vi "Settings Dialog.vi"(8 "error in (no error)":errorcluster, 11 "Settings in":T3={"Connection Configuration"={"Data source"=enum."Serial port", "Connection info"={"VISA resource name"="COM 1", "Baud rate"=9600, "data bits"=8, "stop bits"=0, "parity (0:none)"=enum."None", "flow control (0:none)"=0, "timeout (10sec)"=10000, "termination char\n(0xA = '\\n' = LF) "=10, "Enable Termination\nChar (T)"=TRUE}, "Protocol info"={"Temination char"=255, "Escape char"=254}, "Internet server"={"Web page telemetry"="", "Web page gps"=""}, "Data format"=enum."IDRA data"}, "Logging Configuration"={"Log File Base Path"=path "", "TDMS File Reference"=refnum, "Data format"=enum."IDRA data"}, "Maps config"={"Real-time map config"={"Config path"=path "", "Image path"=path ""}, "Mini map config"={"Config path"=path "", "Image path"=path ""}}, "Data format"=enum."IDRA data"} {"Connection Configuration"."Connection info"."flow control (0:none)" items=["None", "XON/XOFF", "RTS/CTS", "XON/XOFF & RTS/CTS", "DTR/DSR", "XON/XOFF & DTR/DSR"]}) -> (0 "error out":errorcluster, 1 "Cancelled?":bool, 2 "UI Refresh Needed?":bool, 3 "Settings out":T3={"Connection Configuration"={"Data source"=enum."Serial port", "Connection info"={"VISA resource name"="COM 1", "Baud rate"=9600, "data bits"=8, "stop bits"=0, "parity (0:none)"=enum."None", "flow control (0:none)"=0, "timeout (10sec)"=10000, "termination char\n(0xA = '\\n' = LF) "=10, "Enable Termination\nChar (T)"=TRUE}, "Protocol info"={"Temination char"=255, "Escape char"=254}, "Internet server"={"Web page telemetry"="", "Web page gps"=""}, "Data format"=enum."IDRA data"}, "Logging Configuration"={"Log File Base Path"=path "", "TDMS File Reference"=refnum, "Data format"=enum."IDRA data"}, "Maps config"={"Real-time map config"={"Config path"=path "", "Image path"=path ""}, "Mini map config"={"Config path"=path "", "Image path"=path ""}}, "Data format"=enum."IDRA data"} {"Connection Configuration"."Connection info"."flow control (0:none)" items=["None", "XON/XOFF", "RTS/CTS", "XON/XOFF & RTS/CTS", "DTR/DSR", "XON/XOFF & DTR/DSR"]})   [LabVIEW 2015, in "Settings.lvlib"]
doc: "Dialog for selecting user specified settings."
uses:
  Settings.lvlib
  Settings.ctl
  Acquisition/Hardware Configuration.ctl
  Logging/Logging Configuration.ctl
  My Graphs/Gps Map Graph config.ctl
  <vilib>/Utility/xml.llb/Write to XML File(string).vi
  Acquisition/Acquisition.lvlib
  Logging/Logging.lvlib
panel:
  in  "Tab Control":T1(tab)
  in  "Web page gps":string
  in  "Web page telemetry":string
  in  "Data source":T2(ring)
  in  "Baud rate":u32=9600
  in  "Serial port":refnum<visa-resource-name>="COM 1"
  out "Previous data format":enum16{"IDRA data", "XAM data"}(ring)
  in  "Data format":enum16{"IDRA data", "XAM data"}(ring)
  in  "Folder for Log Files":path
  in  "Mini map image (350 x 200)":path
  in  "Configuration path":path
  in  "Big map image (780 x 550)":path
  in  "Cancel Button":bool
  in  "OK Button":bool
  # "Non visible portion of dialog (needed for connector pane)."
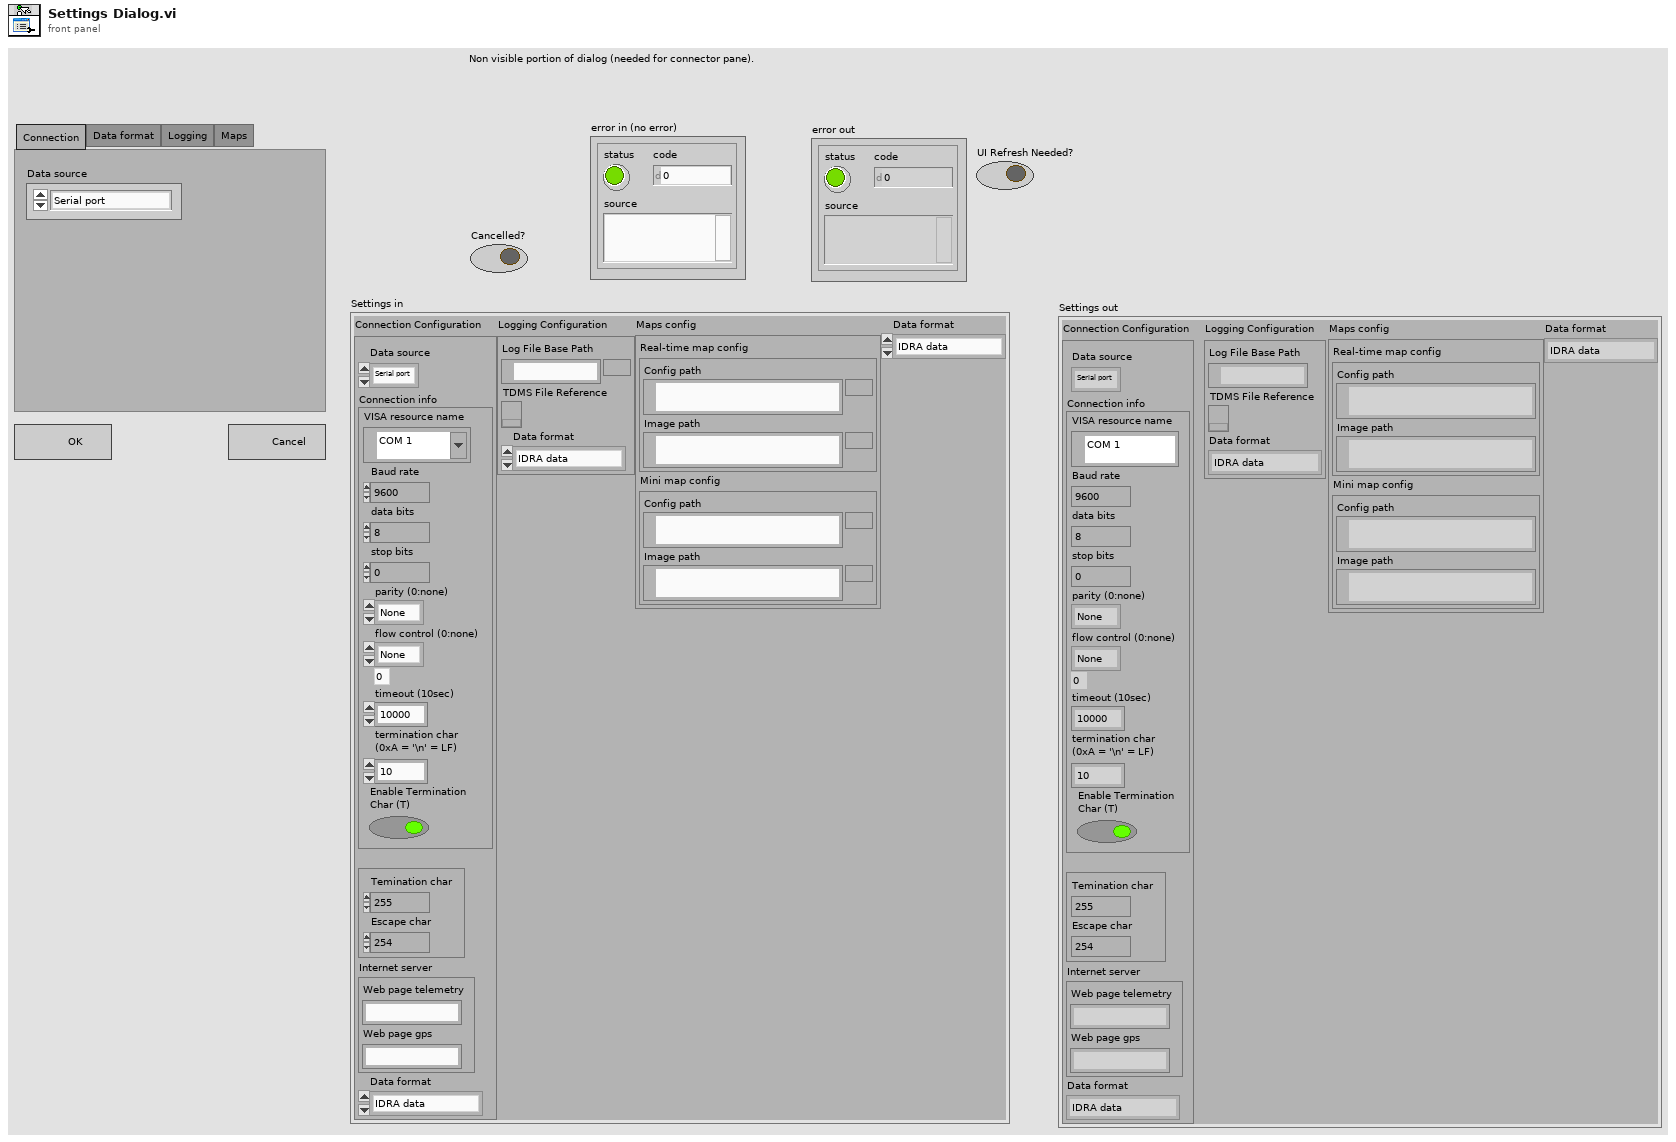
[diagram p1: front panel]
types:
  T1 = enum32{"Connection", "Data format", "Logging", "Maps"}
  T2 = enum16{"Serial port", "Simulated data", "Web page JSON"}
  T3 = typedef "Settings.lvlib/Settings.ctl" = cluster{"Connection Configuration":T4, "Logging Configuration":T5, "Maps config":cluster{"Real-time map config":T6, "Mini map config":T6}, "Data format":enum16{"IDRA data", "XAM data"}}
  T4 = typedef "Acquisition.lvlib/Hardware Configuration.ctl" = cluster{"Data source":enum16{"Serial port", "Simulated data", "Web page JSON"}, "Connection info":cluster{"VISA resource name":refnum<visa-resource-name>, "Baud rate":u32, "data bits":u16, "stop bits":u16, "parity (0:none)":enum16{"None", "Odd", "Even", "Mark", "Space"}, "flow control (0:none)":u16, "timeout (10sec)":u32, "termination char\n(0xA = '\\n' = LF) ":u8, "Enable Termination\nChar (T)":bool}, "Protocol info":cluster{"Temination char":u8, "Escape char":u8}, "Internet server":cluster{"Web page telemetry":string, "Web page gps":string}, "Data format":enum16{"IDRA data", "XAM data"}}
  T5 = typedef "Logging.lvlib/Logging Configuration.ctl" = cluster{"Log File Base Path":path, "TDMS File Reference":refnum<k34>, "Data format":enum16{"IDRA data", "XAM data"}}
  T6 = typedef "Gps Map Graph config.ctl" = cluster{"Config path":path, "Image path":path}
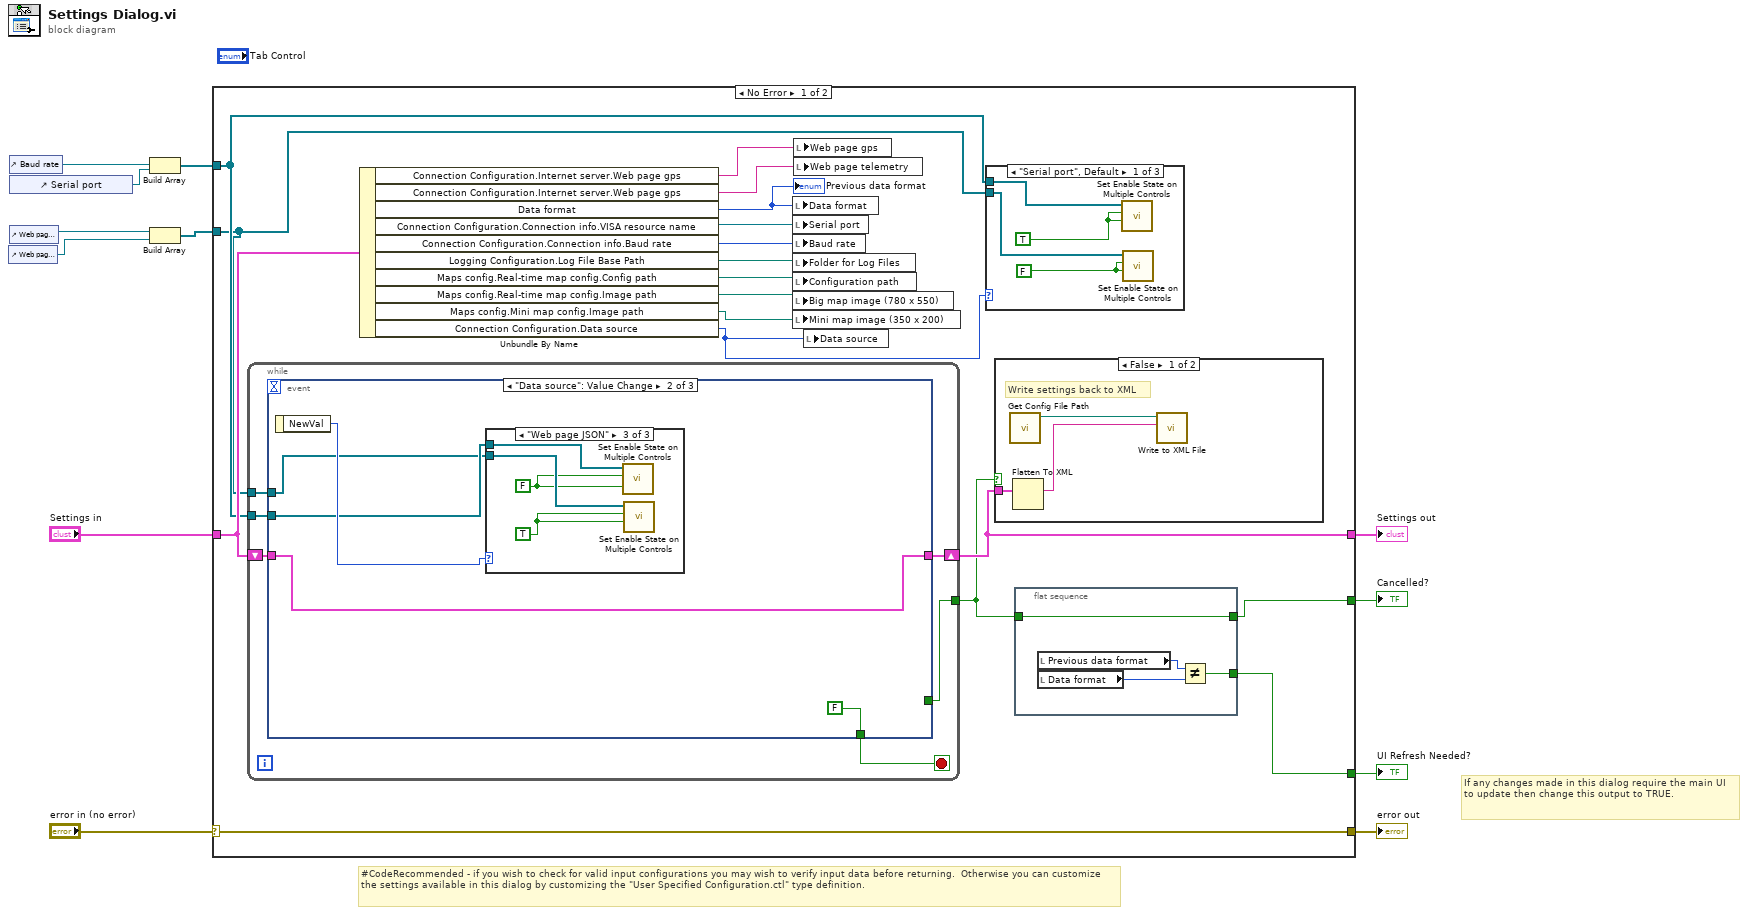
[diagram p0: block diagram]
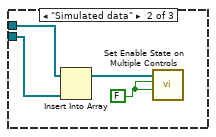
[diagram p2: hidden frame]
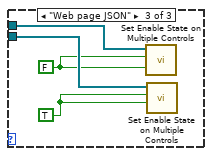
[diagram p3: hidden frame]
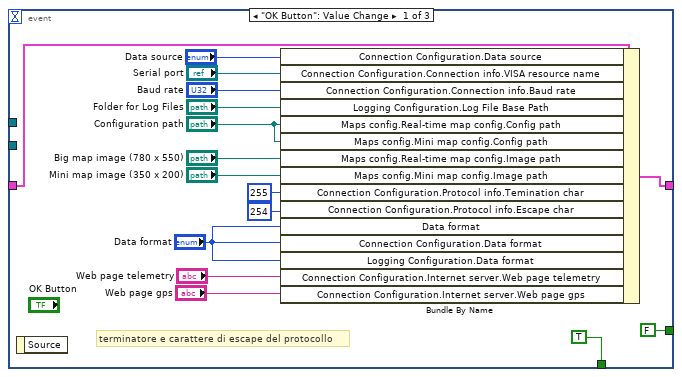
[diagram p4: hidden frame]
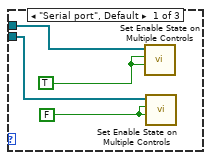
[diagram p5: hidden frame]
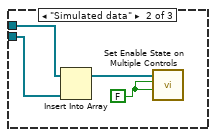
[diagram p6: hidden frame]
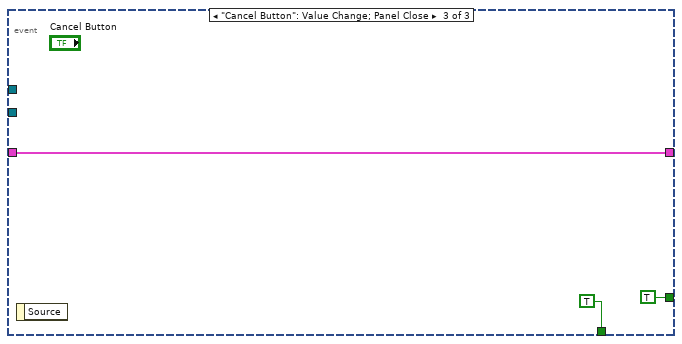
[diagram p7: hidden frame]
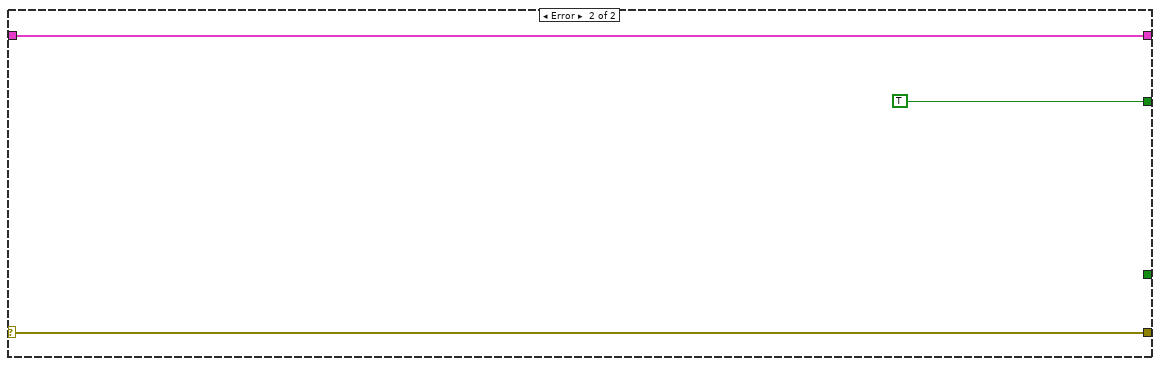
[diagram p9: hidden frame]
diagram:
  # "If any changes made in this dialog require the main UI to update then change this output to TRUE."
  # "#CodeRecommended - if you wish to check for valid input configurations you may wish to verify input data before returning.  Otherwise you can customize the settings available in this dialog by customizing the \"User Specified Configuration.ctl\" type definition."
  n1 = control-ref of="Web page gps"() -> (w1:refnum<vi>)
  n2 = control-ref of="Baud rate"() -> (w5:refnum<vi>)
  n3 = control-ref of="Serial port"() -> (w6:refnum<vi>)
  n4 = control-ref of="Web page telemetry"() -> (w3:refnum<vi>)
  n5 = Build Array(w5, w6) -> (w4:refnum<vi>[])
  n6 = Build Array(w3, w1) -> (w2:refnum<vi>[])
  n7 = case shown="No Error" "error in (no error)" {
    selector: "error in (no error)" -> [w30 w94]
    tunnel: [w30 w94] -> w11
    tunnel: "Settings in" -> [w28 w93]
    tunnel: [w29 w93] -> w9
    tunnel: [w18 _] -> w8
    tunnel: [w16 TRUE ("UI Refresh Needed?")] -> w7
    tunnel: w4 -> [w21 _]
    tunnel: w2 -> [w15 _]
    frame No Error {
      n8 = while {
        tunnel: [w52] -> w17
        shift-right: [w51] -> w29
        shift-left: w28 -> [w50]
        tunnel: w21 -> [w48]
        tunnel: w15 -> [w47]
        stop <- w49 stop-if-true
        n9 = event shown="[1] \"Data source\": Value Change" {
          selector: _ -> [_ _ _]
          dyn-events: _ -> [_ _ _]
          timeout: _ -> [_ _ _]
          tunnel: [w66 w72 w88] -> w51
          tunnel: w50 -> [w67 w72 w88]
          tunnel: [FALSE ("UI Refresh Needed?") _ TRUE ("UI Refresh Needed?")] -> w52
          tunnel: [TRUE FALSE TRUE] -> w49
          tunnel: w48 -> [_ w70 _]
          tunnel: w47 -> [_ w69 _]
          event "OK Button": Value Change {
            # "terminatore e carattere di escape del protocollo"
            n10 = event-data() -> ()  [unwired: 1 in, 1 out]
            n11 = Bundle By Name(cluster=w67, "Connection Configuration.Data source"="Data source", "Connection Configuration.Connection info.VISA resource name"="Serial port", "Connection Configuration.Connection info.Baud rate"="Baud rate", "Logging Configuration.Log File Base Path"="Folder for Log Files", "Maps config.Real-time map config.Config path"="Configuration path", "Maps config.Mini map config.Config path"="Configuration path", "Maps config.Real-time map config.Image path"="Big map image (780 x 550)", "Maps config.Mini map config.Image path"="Mini map image (350 x 200)", "Connection Configuration.Protocol info.Temination char"=u8 255, "Connection Configuration.Protocol info.Escape char"=u8 254, "Data format"="Data format", "Connection Configuration.Data format"="Data format", "Logging Configuration.Data format"="Data format", "Connection Configuration.Internet server.Web page telemetry"="Web page telemetry", "Connection Configuration.Internet server.Web page gps"="Web page gps") -> (w66:T3)
          }
          event "Data source": Value Change {
            n12 = event-data() -> ("NewVal"=w71:T2)  [unwired: 1 in]
            n13 = case shown="\"Web page JSON\"" w71 {
              tunnel: w70 -> [w77 w80 w85]
              tunnel: w69 -> [w74 w79 w84]
              frame "Serial port", Default {
                w75 = FALSE ("Enable?")
                w76 = TRUE ("Enable?")
                n14 = call "Set Enable State on Multiple Controls.vi"("Visible?"=w76, "Enable?"=w76, "Controls"=w77) -> ()  [unwired: 9 in]
                n15 = call "Set Enable State on Multiple Controls.vi"("Visible?"=w75, "Enable?"=w75, "Controls"=w74) -> ()  [unwired: 9 in]
              }
              frame "Simulated data" {
                w81 = FALSE
                n16 = Insert Into Array(array=w80, new element=w79) -> (w78:refnum<vi>[])  [unwired: 1 in]
                n17 = call "Set Enable State on Multiple Controls.vi"("Visible?"=w81, "Enable?"=w81, "Controls"=w78) -> ()  [unwired: 9 in]
              }
              frame "Web page JSON" {
                w82 = TRUE ("Visible?")
                w83 = FALSE ("Visible?")
                n18 = call "Set Enable State on Multiple Controls.vi"("Visible?"=w83, "Enable?"=w83, "Controls"=w85) -> ()  [unwired: 9 in]
                n19 = call "Set Enable State on Multiple Controls.vi"("Visible?"=w82, "Enable?"=w82, "Controls"=w84) -> ()  [unwired: 9 in]
              }
            }
          }
          event "Cancel Button": Value Change; Panel Close {
            n20 = event-data() -> ()  [unwired: 1 in, 1 out]
          }
        }
      }
      n21 = Unbundle By Name(w28) -> ("Connection Configuration.Internet server.Web page gps"=w14:string, "Connection Configuration.Internet server.Web page gps"=w13:string, "Data format"=w19:enum16{"IDRA data", "XAM data"}, "Connection Configuration.Connection info.VISA resource name"=w27:refnum<visa-resource-name>, "Connection Configuration.Connection info.Baud rate"=w26:u32, "Logging Configuration.Log File Base Path"=w25:path, "Maps config.Real-time map config.Config path"=w24:path, "Maps config.Real-time map config.Image path"=w23:path, "Maps config.Mini map config.Image path"=w22:path, "Connection Configuration.Data source"=w20:T2)
      "Previous data format" <- w19
      n22 = local write "Data format"(w19) -> ()
      n23 = local write "Serial port"(w27) -> ()
      n24 = local write "Baud rate"(w26) -> ()
      n25 = local write "Folder for Log Files"(w25) -> ()
      n26 = local write "Configuration path"(w24) -> ()
      n27 = local write "Big map image (780 x 550)"(w23) -> ()
      n28 = local write "Mini map image (350 x 200)"(w22) -> ()
      n29 = local write "Web page gps"(w14) -> ()
      n30 = local write "Web page telemetry"(w13) -> ()
      n31 = local write "Data source"(w20) -> ()
      n32 = case shown="\"Serial port\", Default" w20 {
        tunnel: w21 -> [w34 w37 w42]
        tunnel: w15 -> [w31 w36 w41]
        frame "Serial port", Default {
          w32 = FALSE ("Enable?")
          w33 = TRUE ("Enable?")
          n33 = call "Set Enable State on Multiple Controls.vi"("Visible?"=w33, "Enable?"=w33, "Controls"=w34) -> ()  [unwired: 9 in]
          n34 = call "Set Enable State on Multiple Controls.vi"("Visible?"=w32, "Enable?"=w32, "Controls"=w31) -> ()  [unwired: 9 in]
        }
        frame "Simulated data" {
          w38 = FALSE
          n35 = Insert Into Array(array=w37, new element=w36) -> (w35:refnum<vi>[])  [unwired: 1 in]
          n36 = call "Set Enable State on Multiple Controls.vi"("Visible?"=w38, "Enable?"=w38, "Controls"=w35) -> ()  [unwired: 9 in]
        }
        frame "Web page JSON" {
          w39 = TRUE ("Visible?")
          w40 = FALSE ("Visible?")
          n37 = call "Set Enable State on Multiple Controls.vi"("Visible?"=w40, "Enable?"=w40, "Controls"=w42) -> ()  [unwired: 9 in]
          n38 = call "Set Enable State on Multiple Controls.vi"("Visible?"=w39, "Enable?"=w39, "Controls"=w41) -> ()  [unwired: 9 in]
        }
      }
      n39 = case shown="False" w17 {
        tunnel: w29 -> [w90 _]
        frame False {
          # "Write settings back to XML"
          n40 = call "Get Config File Path.vi"() -> ("XML File Path"=w91:path)  [unwired: 10 in, 1 out]
          n41 = Flatten To XML(anything=w90) -> (xml string=w89:string)
          n42 = call-poly <vilib>:"Write to XML File.vi"("XML Input"=w89, "XML File Path"=w91) -> ()  [unwired: 7 in, 3 out]
        }
        frame True {
        }
      }
      n43 = flat-sequence {
        tunnel: [w44] -> w18
        tunnel: w17 -> [w43]
        tunnel: [w43] -> w16
        frame #0 {
          n44 = local read "Previous data format"() -> (w46:enum16{"IDRA data", "XAM data"})
          n45 = local read "Data format"() -> (w45:enum16{"IDRA data", "XAM data"})
          n46 = Not Equal?(x=w46, y=w45) -> (x != y?=w44:bool)
        }
      }
    }
    frame Error {
    }
  }
  "UI Refresh Needed?" <- w8
  "error out" <- w11
  "Settings out" <- w9
  "Cancelled?" <- w7
